vi "example 1.vi"() -> ()   [LabVIEW 2015]
panel:
  out "Numeric":dbl
  out "Waveform Graph":dynamicdata(graph)
  out "Meter":dbl(knob) scale=0.0..10.0
  in  "stop":bool
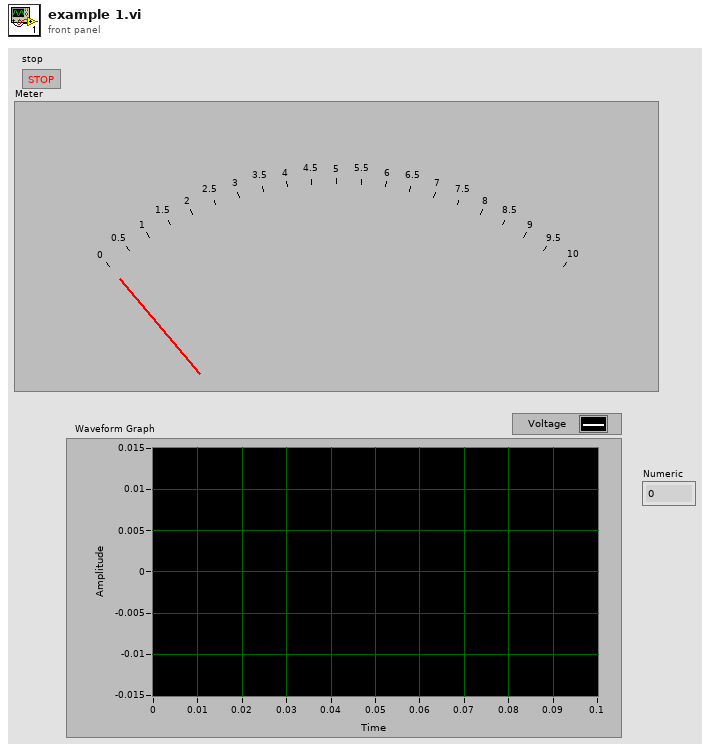
[diagram p1: front panel]
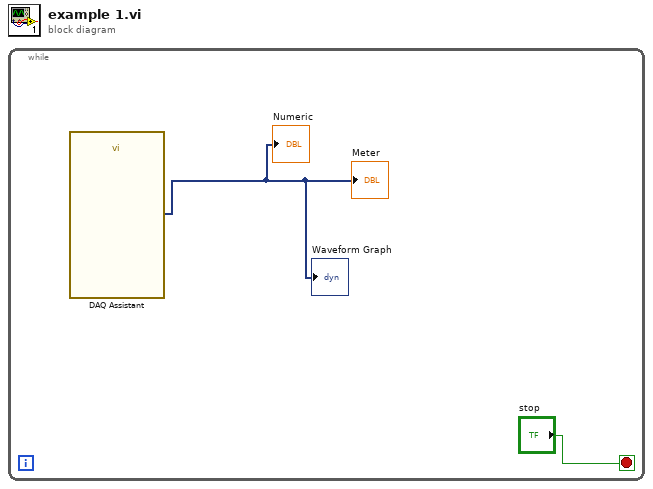
[diagram p0: block diagram]
diagram:
  n1 = while {
    stop <- "stop" stop-if-true
    n2 = call "DAQ Assistant"() -> ("data"=→"Meter" →"Waveform Graph" →"Numeric":dynamicdata)  [unwired: 16 in, 3 out]
  }
